vi "Proba3.vi"() -> ()   [LabVIEW 2013]
uses:
  Parameterek.ctl
panel:
  out "Q_belsolevego":dbl[](graph)
  out "T_belsolevego":dbl[](graph)
  out "T_belso":dbl[][](graph)
  out "Q_belso":dbl[][](graph)
  out "T_kulso":dbl[][](graph)
  out "Q_kulso":dbl[][](graph)
  in  "Parameterek":T1={"rholevego"=0.0, "Vlevego"=0.0, "Mlevego"=0.0, "clevego"=0.0, "rho PCM"=1100.0, "rho kulso"=28.3, "Dkulso"=0.1, "nkulso"=10, "dkulso"=0.0, "vkulso"=0.0, "rho kozepso"=28.3, "Dkozepso"=0.06, "nkozepso"=6, "dkozepso"=0.0, "vkozepso"=0.0, "mkozepso"=0.0, "mkulso"=0.0, "rho belso"=28.3, "Dbelso"=0.1, "nbelso"=10, "dbelso"=0.0, "vbelso"=0.0, "mbelso"=0.0, "Xpcm_kulso"=0.3, "Xpcm_belso"=0.3, "mpcm_kulso"=0.0, "mpcm_belso"=0.0, "mkulso_pcm"=0.0, "mbelso_pcm"=0.0, "ckulso"=1.13, "ckozepso"=1.13, "cbelso"=1.13, "cpcm_szilard"=1.9, "cpcm_foly"=1.5, "ckulso_Topalatt"=0.0, "cbelso_Topalatt"=0.0, "ckulso_Topfelett"=0.0, "cbelso_Topfelett"=0.0, "hpcm_olv"=140.0, "ckulso_eff_Tolv"=0.0, "cbelso_eff_Tolv"=0.0, "Qkulso_op_also"=0.0, "Qkulso_op_felso"=0.0, "Qbelso_op_also"=0.0, "Qbelso_op_felso"=0.0, "lambda_kulso"=5e-05, "lambda_kozepso"=5e-05, "lambda_belso"=5e-05, "lambda_pcm"=0.00018, "VXpcm_kulso"=0.0, "VXpcm_belso"=0.0, "lambda_kulsoPCM"=0.0, "lambda_belsoPCM"=0.0, "Alfa_kulso"=0.015, "Alfa_belso"=0.006, "Alfa_kont"=0.03, "Top_also"=24.0, "Top_felso"=28.0, "cpcm_olvnelkul"=0.0, "Tbelsolevego_0"=22.0}
  out "T_kozepso":dbl[][](graph)
  out "T_kulsolevego":dbl[](graph)
  out "Q_kozepso":dbl[][](graph)
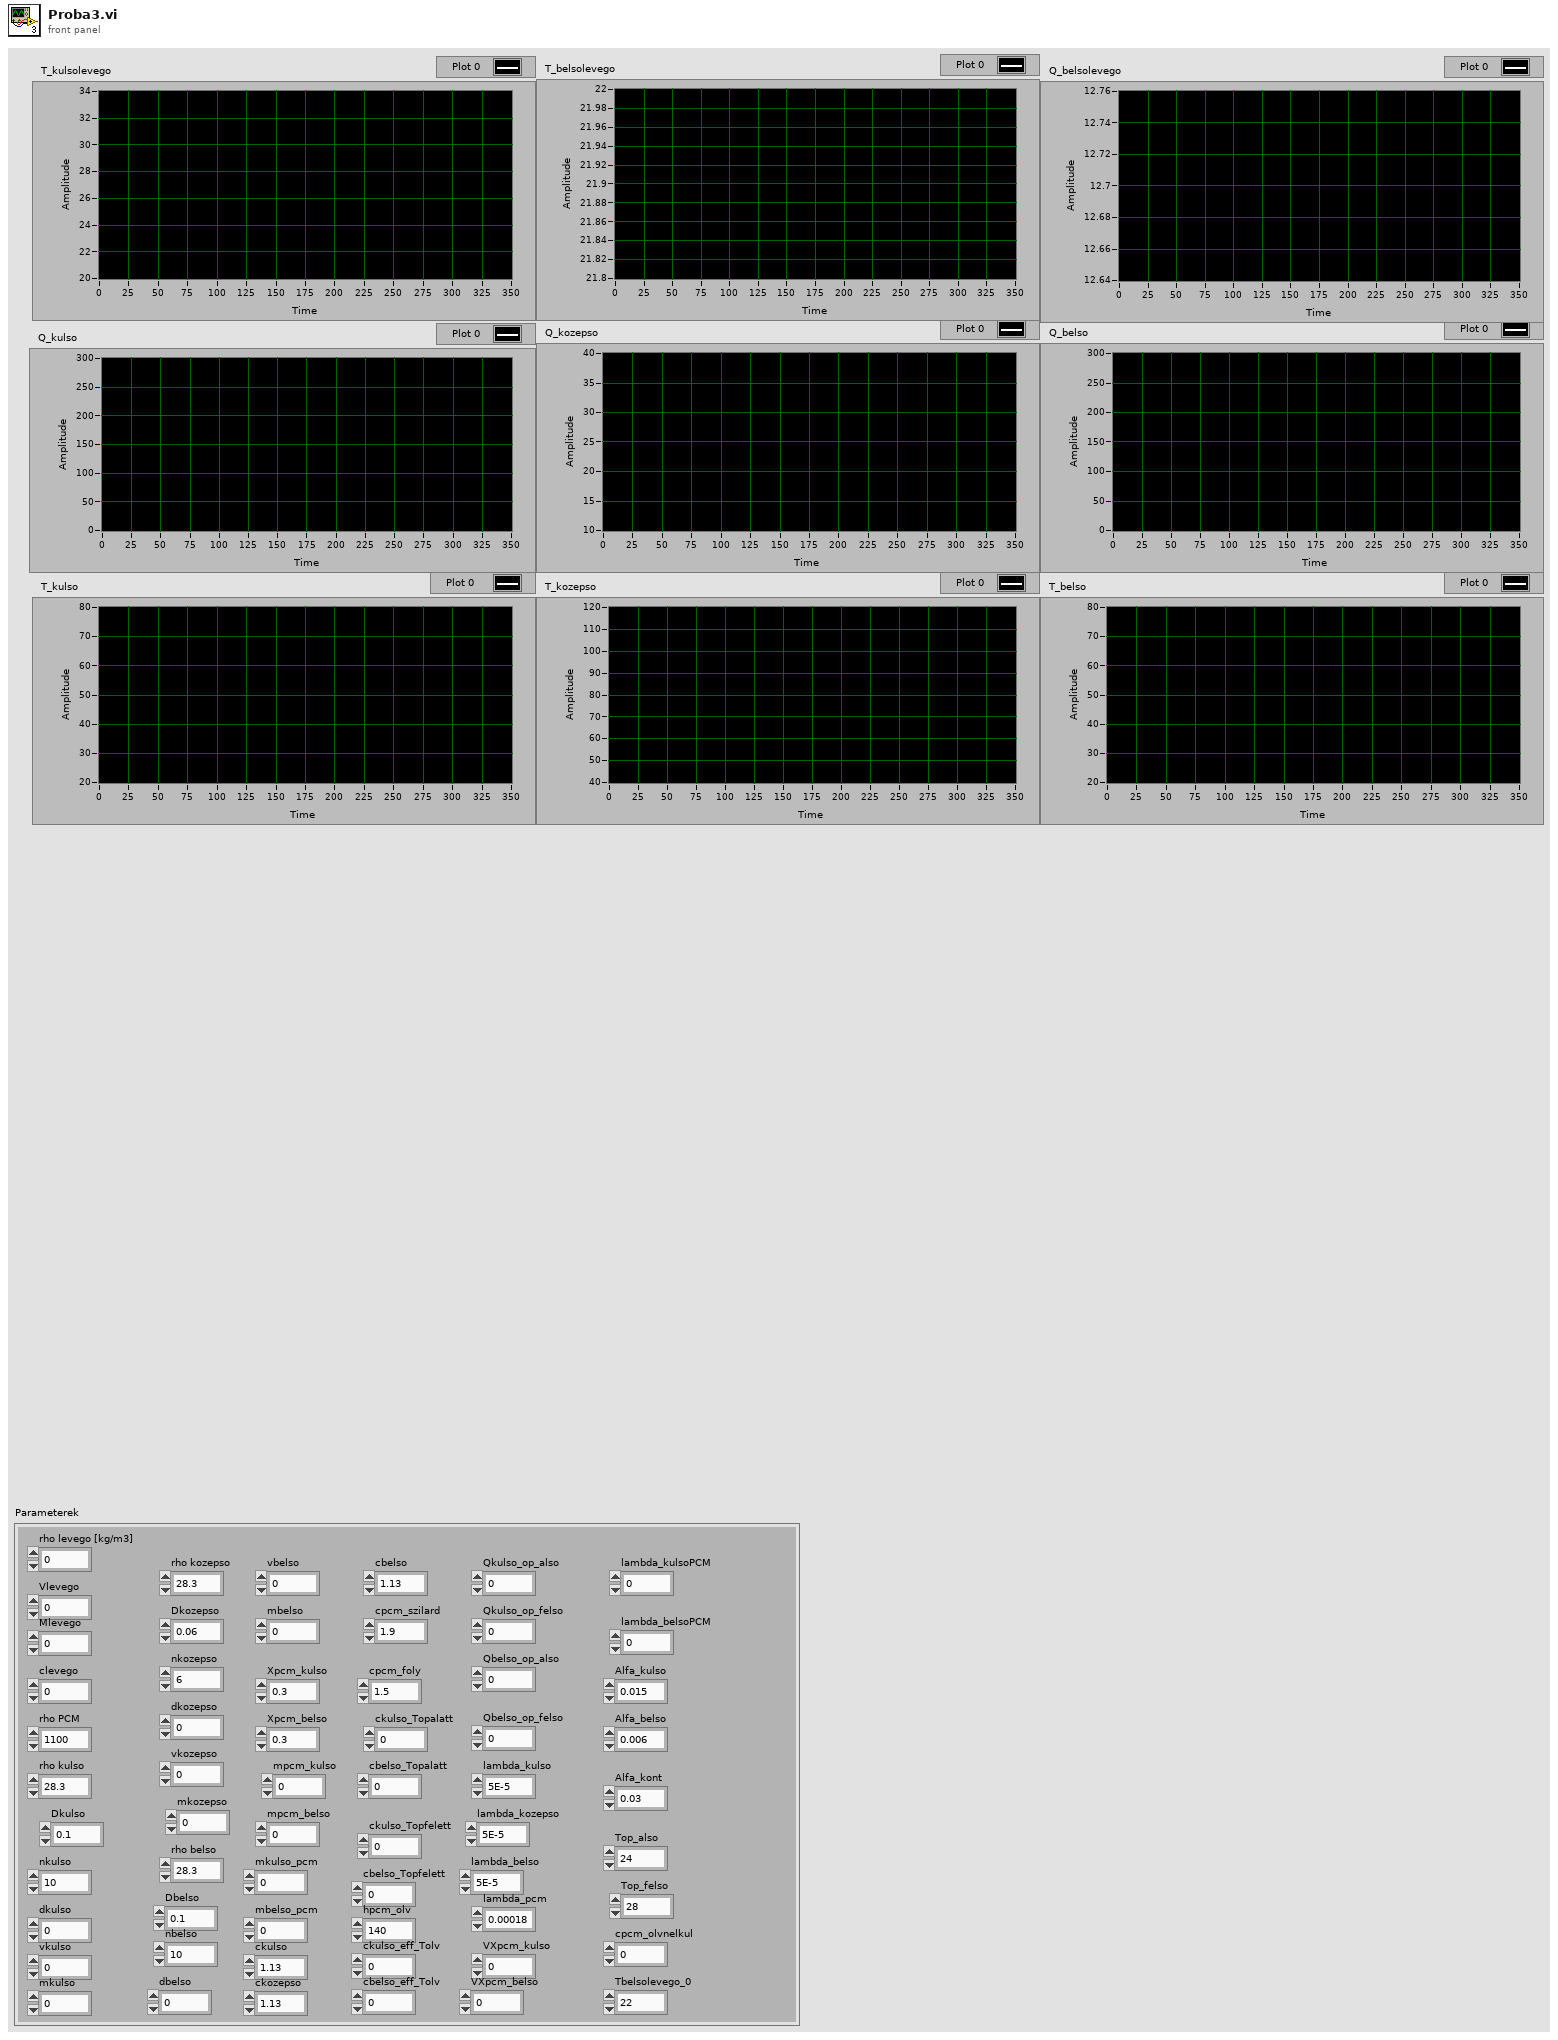
[diagram p1: front panel]
types:
  T1 = typedef "Parameterek.ctl" = cluster{"rholevego":dbl, "Vlevego":dbl, "Mlevego":dbl, "clevego":dbl, "rho PCM":dbl, "rho kulso":dbl, "Dkulso":dbl, "nkulso":i32, "dkulso":dbl, "vkulso":dbl, "rho kozepso":dbl, "Dkozepso":dbl, "nkozepso":i32, "dkozepso":dbl, "vkozepso":dbl, "mkozepso":dbl, "mkulso":dbl, "rho belso":dbl, "Dbelso":dbl, "nbelso":i32, "dbelso":dbl, "vbelso":dbl, "mbelso":dbl, "Xpcm_kulso":dbl, "Xpcm_belso":dbl, "mpcm_kulso":dbl, "mpcm_belso":dbl, "mkulso_pcm":dbl, "mbelso_pcm":dbl, "ckulso":dbl, "ckozepso":dbl, "cbelso":dbl, "cpcm_szilard":dbl, "cpcm_foly":dbl, "ckulso_Topalatt":dbl, "cbelso_Topalatt":dbl, "ckulso_Topfelett":dbl, "cbelso_Topfelett":dbl, "hpcm_olv":dbl, "ckulso_eff_Tolv":dbl, "cbelso_eff_Tolv":dbl, "Qkulso_op_also":dbl, "Qkulso_op_felso":dbl, "Qbelso_op_also":dbl, "Qbelso_op_felso":dbl, "lambda_kulso":dbl, "lambda_kozepso":dbl, "lambda_belso":dbl, "lambda_pcm":dbl, "VXpcm_kulso":dbl, "VXpcm_belso":dbl, "lambda_kulsoPCM":dbl, "lambda_belsoPCM":dbl, "Alfa_kulso":dbl, "Alfa_belso":dbl, "Alfa_kont":dbl, "Top_also":dbl, "Top_felso":dbl, "cpcm_olvnelkul":dbl, "Tbelsolevego_0":dbl}
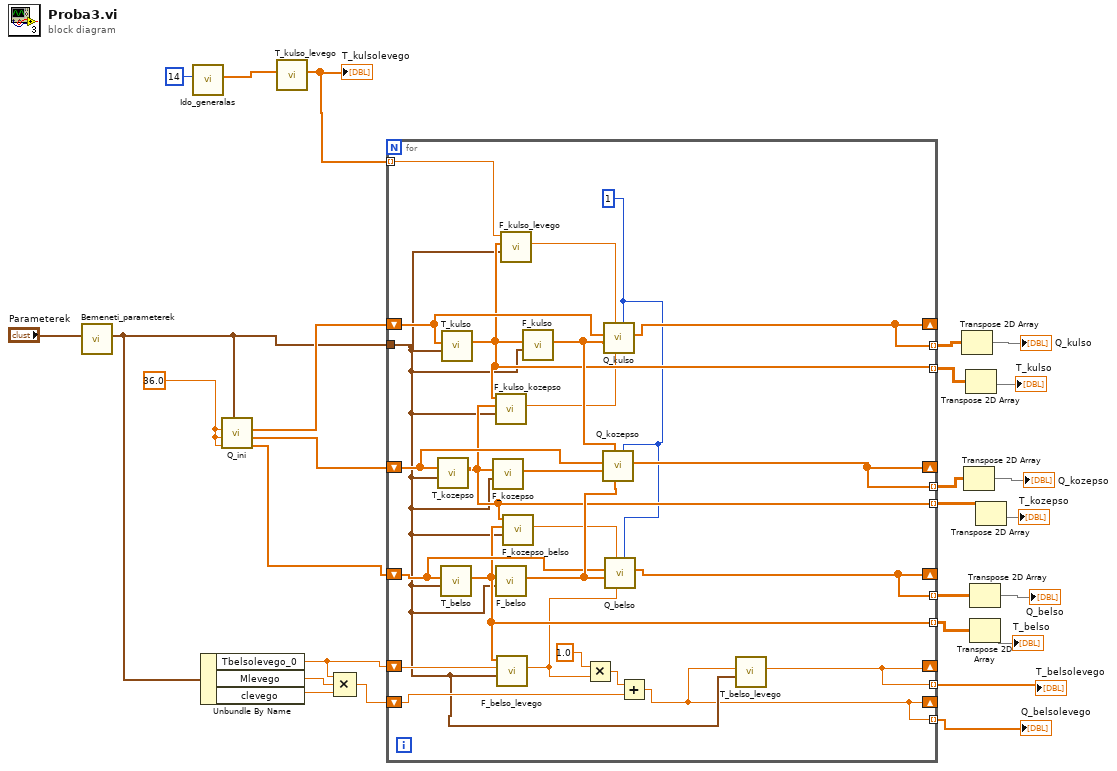
[diagram p0: block diagram]
diagram:
  w12 = 36.0 ("Q_kulso_0")
  n1 = call "Bemeneti_parameterek.vi"("Parameterek"="Parameterek") -> ("Parameterek 2"=w4:T1)  [unwired: 10 in]
  n2 = call "Ido_generalas.vi"("t_sim [nap]"=14) -> ("t_vektor"=w27:dbl[])  [unwired: 10 in]
  n3 = Unbundle By Name(w4) -> ("Tbelsolevego_0"=w5:dbl, "Mlevego"=w3:dbl, "clevego"=w2:dbl)
  n4 = call "Q_ini.vi"("Parameterek"=w4, "Q_belso_0"=w12, "Q_kozepso_0"=w12, "Q_kulso_0"=w12) -> ("Q_belso_0_vektor"=w9:dbl[], "Q_kozepso_0_vektor"=w10:dbl[], "Q_kulso_0 vektor"=w11:dbl[])  [unwired: 5 in]
  n5 = call "T_kulso_levego.vi"("t_vektor"=w27) -> ("T_kulso_levego_vektor"=w26:dbl[])  [unwired: 9 in, 1 out]
  "T_kulsolevego" <- w26
  n6 = Compound Arithmetic op=MULTIPLY(w5, w3, w2) -> (w6:dbl)
  n7 = for {
    tunnel: w26 -> [w51] mode=indexing
    shift-right: [w50] -> _
    shift-left: w10 -> [w52]
    tunnel: [w50] -> w25 mode=indexing
    tunnel: [w39] -> w22 mode=indexing
    tunnel: w4 -> [w31]
    shift-right: [w46] -> _
    shift-left: w11 -> [w49]
    shift-right: [w43] -> _
    shift-left: w9 -> [w44]
    tunnel: [w46] -> w19 mode=indexing
    tunnel: [w40] -> w17 mode=indexing
    tunnel: [w43] -> w15 mode=indexing
    tunnel: [w37] -> w13 mode=indexing
    shift-right: [w30] -> _
    shift-left: w5 -> [w36]
    shift-right: [w28] -> _
    shift-left: w6 -> [w35]
    tunnel: [w30] -> w7 mode=indexing
    tunnel: [w28] -> w1 mode=indexing
    w32 = 1
    n8 = call "T_kozepso.vi"("Parameterek"=w31, "Q kozepso vektor"=w52) -> ("T kozepso vektor"=w39:dbl[])  [unwired: 9 in]
    n9 = call "T_belso.vi"("Parameterek"=w31, "Q belso vektor"=w44) -> ("T belso vektor"=w37:dbl[])  [unwired: 9 in]
    n10 = call "T_kulso.vi"("Parameterek"=w31, "Q kulso vektor"=w49) -> ("T kulso vektor"=w40:dbl[])  [unwired: 9 in]
    n11 = call "F_kozepso.vi"("Parameterek"=w31, "T_kozepso_vektor"=w39) -> ("F_kozepso_vektor"=w41:dbl[])  [unwired: 9 in]
    n12 = call "F_kulso_kozepso.vi"("T_kulso_vektor"=w40, "T_kozepso_vektor"=w39, "Parameterek"=w31) -> ("F_10_11"=w38:dbl)  [unwired: 7 in]
    n13 = call "F_belso.vi"("Parameterek"=w31, "T_belso_vektor"=w37) -> ("F_belso_vektor"=w45:dbl[])  [unwired: 9 in]
    n14 = call "F_belso_levego.vi"("Parameterek"=w31, "T_belso_levego"=w36, "T_belso_vektor"=w37) -> ("F_fal_belso_levego"=w33:dbl)  [unwired: 8 in]
    n15 = call "F_kulso_levego.vi"("Parameterek"=w31, "T_kulso_vektor"=w40, "T_kulso_levego"=w51) -> ("F_kulso_levego_fal"=w47:dbl)  [unwired: 8 in]
    n16 = call "F_kozepso_belso.vi"("T_kozepso_vektor"=w39, "T_belso_vektor"=w37, "Parameterek"=w31) -> ("F_16_17"=w42:dbl)  [unwired: 7 in]
    n17 = call "F_kulso.vi"("Parameterek"=w31, "T_kulso_vektor"=w40) -> ("F_kulso_vektor"=w48:dbl[])  [unwired: 9 in]
    n18 = Multiply(x=1.0, y=w33) -> (x*y=w34:dbl)
    n19 = call "Q_kozepso.vi"("idolepes"=w32, "F_belso_vektor"=w45, "F_kulso_vektor"=w48, "F_kozepso_vektor"=w41, "Q_kozepso_elozo_vektor"=w52) -> ("Q_kozepso_aktualis_vektor"=w50:dbl[])  [unwired: 6 in]
    n20 = call "Q_kulso.vi"("idolepes"=w32, "F_10_11"=w38, "F_kulso_levego_fal"=w47, "F_kulso_vektor"=w48, "Q_kulso_elozo_vektor"=w49) -> ("Q_kulso_aktualis_vektor"=w46:dbl[])  [unwired: 6 in]
    n21 = call "Q_belso.vi"("idolepes"=w32, "F_belso_fal"=w33, "F_16_17"=w42, "F_belso_vektor"=w45, "Q_belso_elozo_vektor"=w44) -> ("Q_belso_aktualis_vektor"=w43:dbl[])  [unwired: 6 in]
    n22 = Add(x=w34, y=w35) -> (x+y=w28:dbl)
    n23 = call "T_belso_levego.vi"("Parameterek"=w31, "Q_belsolevego"=w28) -> ("T_belsolevego"=w30:dbl)  [unwired: 9 in]
  }
  "T_belsolevego" <- w7
  "Q_belsolevego" <- w1
  n24 = Transpose 2D Array(2D array=w19) -> (transposed array=→"Q_kulso":dbl[][])
  n25 = Transpose 2D Array(2D array=w25) -> (transposed array=→"Q_kozepso":dbl[][])
  n26 = Transpose 2D Array(2D array=w17) -> (transposed array=→"T_kulso":dbl[][])
  n27 = Transpose 2D Array(2D array=w15) -> (transposed array=→"Q_belso":dbl[][])
  n28 = Transpose 2D Array(2D array=w13) -> (transposed array=→"T_belso":dbl[][])
  n29 = Transpose 2D Array(2D array=w22) -> (transposed array=→"T_kozepso":dbl[][])
